vi "Scanner.vi"() -> ()   [LabVIEW 2013]
uses:
  Database/Database.lvclass
  Image/Image.lvclass
panel:
  in  "Tab Control":T1(tab)
  out "Image":T2(plugin-control)
  in  "Scan Properties":T3={"X Size"=512.0, "Y Size"=512.0, "lens"=20.0, "mag"=1.0, "Angle"=0.0}
  in  "Session":path=path "Z:/users/Manolis/Labview/Scanner/sessions_Win7.dsn"
  in  "stop":bool
  in  "x corrector":dbl=1.0
  in  "y corrector":dbl=1.0
  in  "condition":string
  out "Scan Clusters":T4(array[cluster])
  out "Vessel Cluster":T5
  out "iDatabase":i32
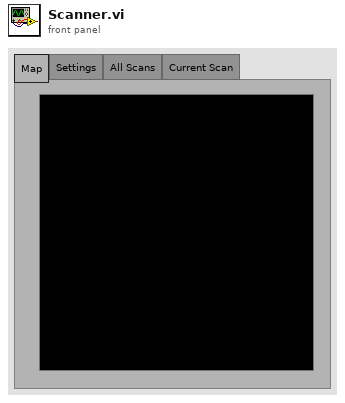
[diagram p1: front panel]
types:
  T1 = enum32{"Map", "Settings", "All Scans", "Current Scan"}
  T2 = typedef "IMAQ Image.ctl" = refnum<image>
  T3 = cluster{"X Size":dbl, "Y Size":dbl, "lens":dbl, "mag":dbl, "Angle":dbl}
  T4 = cluster{"scan_idx":string, "lens":string, "mag":string, "x":string, "y":string, "z":string, "scan_rotation":string, "scan_prog":string}[]
  T5 = cluster{"scan_idx":i32, "lens":i32, "mag":dbl, "x":dbl, "y":dbl, "mouse_id":i32, "exp_date":string, "file_name":string, "file_path":path}
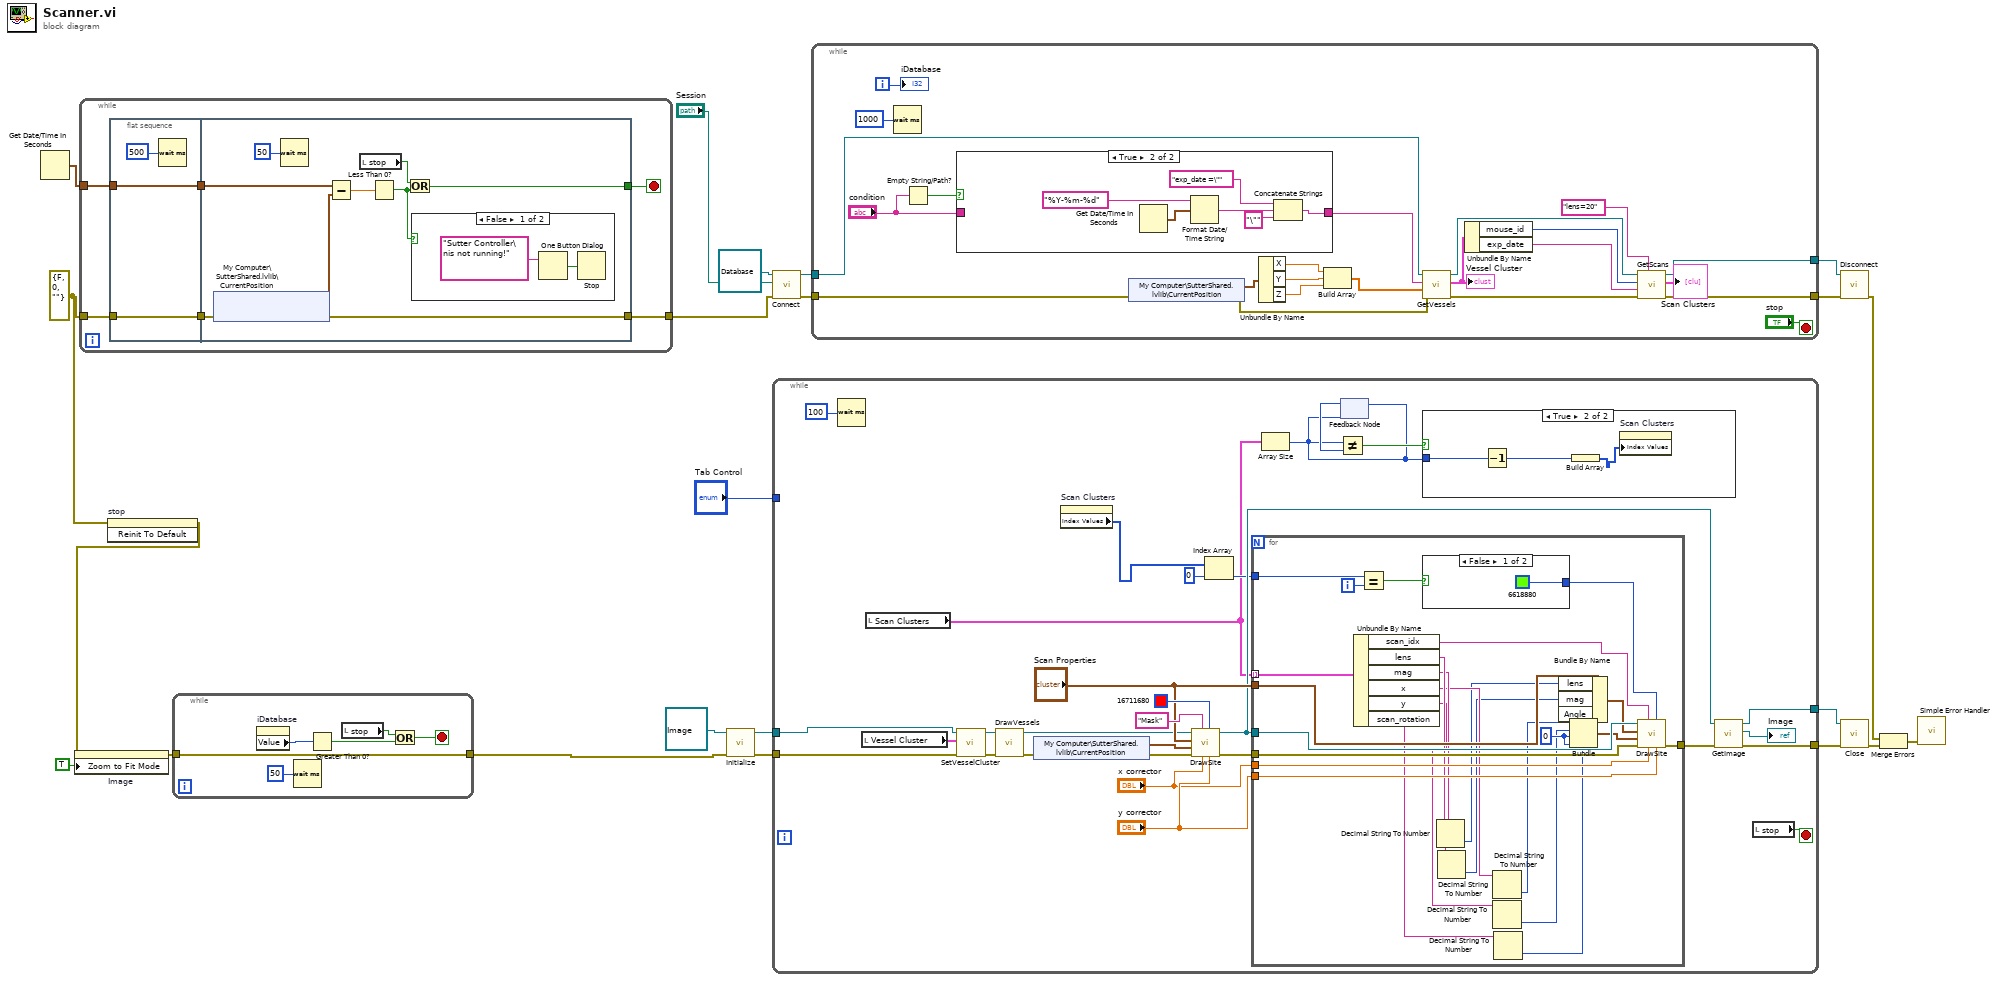
[diagram p0: block diagram]
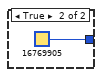
[diagram p4: hidden frame]
diagram:
  w3 = errorcluster {"status"=FALSE, "code"=0, "source"=""} ("error in (no error)")
  n1 = Get Date/Time In Seconds() -> (seconds since 1Jan1904=w5:timestamp)
  n2 = while {
    tunnel: w3 -> [w27]
    tunnel: [w26] -> w7
    tunnel: w5 -> [w25]
    stop <- w28 stop-if-true
    n3 = flat-sequence {
      tunnel: w25 -> [w30]
      tunnel: w27 -> [w31]
      tunnel: [w31] -> w24
      tunnel: [w30] -> w23
      tunnel: [w39] -> w28
      tunnel: [w36] -> w26
      tunnel: w24 -> [w37]
      tunnel: w23 -> [w34]
      frame #0 {
        n4 = Wait (ms)(milliseconds to wait=u32 500) -> ()  [unwired: 1 out]
      }
      frame #1 {
        n5 = shared-variable "My Computer\\SutterShared.lvlib\\CurrentPosition"(error in=w37) -> (error out=w36:errorcluster, w35:timestamp)  [unwired: 1 out]
        n6 = Wait (ms)(milliseconds to wait=u32 50) -> ()  [unwired: 1 out]
        n7 = Subtract(x=w34, y=w35) -> (x-y=w33:dbl)
        n8 = local read "stop"() -> (w38:bool)
        n9 = Less Than 0?(x=w33) -> (x < 0?=w32:bool)
        n10 = Or(x=w38, y=w32) -> (x .or. y?=w39:bool)
        n11 = case shown="False" w32 {
          frame False {
            n12 = One Button Dialog(message="Sutter Controller\nis not running!") -> (true=w41:bool)  [unwired: 1 in]
            n13 = Stop(stop? (T)=w41) -> ()
          }
          frame True {
          }
        }
      }
    }
  }
  n14 = invoke on="stop" class="Bool (strict)" method="Reinit To Default"(error in=w3) -> (error out=w2:errorcluster)  [unwired: 2 in, 2 out]
  n15 = property on="Image" class="ImageControl"(error in=w2, "Zoom to Fit Mode"=TRUE) -> (error out=w9:errorcluster)  [unwired: 1 in, 1 out]
  n16 = while {
    tunnel: w9 -> [w46]
    tunnel: [w46] -> w8
    stop <- w43 stop-if-true
    n17 = property on="iDatabase" class="DigNum (strict)"() -> ("Value"=w48:i32)  [unwired: 2 in, 2 out]
    n18 = Wait (ms)(milliseconds to wait=u32 50) -> ()  [unwired: 1 out]
    n19 = Greater Than 0?(x=w48) -> (x > 0?=w45:bool)
    n20 = local read "stop"() -> (w44:bool)
    n21 = Or(x=w44, y=w45) -> (x .or. y?=w43:bool)
  }
  n22 = call-dynamic "Initialize.vi"("error in (no error)"=w8, "Image in"=refnum<class "Image.lvclass"> refnum) -> ("error out"=w12:errorcluster, "Image out"=w13:refnum<class "Image.lvclass">)  [unwired: 8 in]
  n23 = call-dynamic "Connect.vi"("error in (no error)"=w7, "Session"="Session", "Database in"=refnum<class "Database.lvclass"> refnum) -> ("error out"=w19:errorcluster, "Database out"=w22:refnum<class "Database.lvclass">)  [unwired: 7 in]
  n24 = while {
    tunnel: w13 -> [w76]
    tunnel: w12 -> [w75]
    tunnel: [w74] -> w11
    tunnel: [w73] -> w10
    tunnel: "Tab Control" -> [_]
    stop <- w77 stop-if-true
    n25 = Wait (ms)(milliseconds to wait=u32 100) -> ()  [unwired: 1 out]
    n26 = local read "Vessel Cluster"() -> (w67:T5)
    n27 = local read "Scan Clusters"() -> (w57:T4)
    n28 = call-dynamic "SetVesselCluster.vi"("error in (no error)"=w75, "Vessel Cluster"=w67, "Image in"=w76) -> ("error out"=w66:errorcluster, "Image out"=w72:refnum<class "Image.lvclass">)  [unwired: 7 in]
    n29 = call-dynamic "DrawVessels.vi"("error in (no error)"=w66, "Image in"=w72) -> ("error out"=w52:errorcluster, "Image out"=w65:refnum<class "Image.lvclass">)  [unwired: 8 in]
    n30 = shared-variable "My Computer\\SutterShared.lvlib\\CurrentPosition"(error in=w52) -> (w53:cluster{"X":dbl, "Y":dbl, "Z":dbl, "Depth":dbl}, error out=w51:errorcluster)
    n31 = property on="Scan Clusters" class="Arr (strict)"() -> ("Index Values"=w50:u32[])  [unwired: 2 in, 2 out]
    n32 = call-dynamic "DrawSite.vi"("y corrector"="y corrector", "Color"=u32 16711680, "x corrector"="x corrector", "Group"="Mask", "error in (no error)"=w51, "Position"=w53, "Scan Properties"="Scan Properties", "Image in"=w65) -> ("error out"=w63:errorcluster, "Image out"=w64:refnum<class "Image.lvclass">)  [unwired: 2 in]
    n33 = Index Array(array=w50, index=0) -> (element=w58:u32)
    n34 = for {
      tunnel: w64 -> [w105]
      tunnel: w57 -> [w104] mode=indexing
      tunnel: "Scan Properties" -> [w103]
      tunnel: w63 -> [w100]
      tunnel: [w99] -> w62
      tunnel: "y corrector" -> [w98]
      tunnel: "x corrector" -> [w97]
      tunnel: w58 -> [w95]
      i -> [w96]
      w92 = 0
      n35 = Unbundle By Name(w104) -> ("scan_idx"=w91:string, "lens"=w90:string, "mag"=w89:string, "x"=w88:string, "y"=w87:string, "scan_rotation"=w86:string)
      n36 = Equal?(x=w95, y=w96) -> (x = y?=w94:bool)
      n37 = case shown="False" w94 {
        tunnel: [u32 6618880 ("Color") u32 16769905 ("Color")] -> w93
        frame False {
        }
        frame True {
        }
      }
      n38 = Decimal String To Number(string=w90) -> (number=w85:i32)  [unwired: 2 in, 1 out]
      n39 = Decimal String To Number(string=w89) -> (number=w84:i32)  [unwired: 2 in, 1 out]
      n40 = Decimal String To Number(string=w88) -> (number=w82:i32)  [unwired: 2 in, 1 out]
      n41 = Decimal String To Number(string=w87) -> (number=w81:i32)  [unwired: 2 in, 1 out]
      n42 = Decimal String To Number(string=w86) -> (number=w83:i32)  [unwired: 2 in, 1 out]
      n43 = Bundle By Name(cluster=w103, "lens"=w85, "mag"=w84, "Angle"=w83) -> (w102:T3)
      n44 = Bundle(w82, w81, w92, w92) -> (w101:cluster{i32, i32, i32, i32})  [unwired: 1 in]
      n45 = call-dynamic "DrawSite.vi"("y corrector"=w98, "Color"=w93, "x corrector"=w97, "Group"=w91, "error in (no error)"=w100, "Position"=w101, "Scan Properties"=w102, "Image in"=w105) -> ("error out"=w99:errorcluster)  [unwired: 2 in, 1 out]
    }
    n46 = Array Size(array=w57) -> (size(s)=w54:i32)
    n47 = feedback-in #1(w54) -> ()
    n48 = feedback #1(w54) -> (w56:i32)
    n49 = Not Equal?(x=w54, y=w56) -> (x != y?=w55:bool)
    n50 = case shown="True" w55 {
      tunnel: w54 -> [_ w80]
      frame False {
      }
      frame True {
        n51 = Decrement(x=w80) -> (x-1=w79:i32)
        n52 = Build Array(w79) -> (w78:i32[])
        n53 = property on="Scan Clusters" class="Arr (strict)"("Index Values"=w78) -> ()  [unwired: 2 in, 2 out]
      }
    }
    n54 = call-dynamic "GetImage.vi"("error in (no error)"=w62, "Image in"=w64) -> ("error out"=w73:errorcluster, "Image"=→"Image":T2, "Image out"=w74:refnum<class "Image.lvclass">)  [unwired: 7 in]
    n55 = local read "stop"() -> (w77:bool)
  }
  n56 = while {
    tunnel: w22 -> [w130]
    tunnel: [w129] -> w20
    tunnel: w19 -> [w116]
    tunnel: [w128] -> w18
    i -> [w117]
    stop <- "stop" stop-if-true
    n57 = Wait (ms)(milliseconds to wait=u32 1000) -> ()  [unwired: 1 out]
    n58 = Empty String/Path?(string/path="condition") -> (empty?=w126:bool)
    n59 = case shown="True" w126 {
      tunnel: [w131 w135] -> w124
      tunnel: "condition" -> [w131 _]
      frame False {
      }
      frame True {
        n60 = Get Date/Time In Seconds() -> (seconds since 1Jan1904=w134:timestamp)
        n61 = Format Date/Time String(time format string (%c)="%Y-%m-%d", seconds (now)=w134) -> (date/time string=w132:string)  [unwired: 1 in]
        n62 = Concatenate Strings("exp_date =\"", w132, "\"" ("string")) -> (w135:string)
      }
    }
    n63 = shared-variable "My Computer\\SutterShared.lvlib\\CurrentPosition"(error in=w116) -> (w113:cluster{"X":dbl, "Y":dbl, "Z":dbl, "Depth":dbl}, error out=w115:errorcluster)
    n64 = Unbundle By Name(w113) -> ("X"=w112:dbl, "Y"=w111:dbl, "Z"=w110:dbl)
    n65 = Build Array(w112, w111, w110) -> (w109:dbl[])
    n66 = call-dynamic "GetVessels.vi"("error in (no error)"=w115, "Position"=w109, "condition"=w124, "Database in"=w130) -> ("error out"=w122:errorcluster, "Vessel Cluster"=w119:T5, "Database out"=w123:refnum<class "Database.lvclass">)  [unwired: 5 in]
    "Vessel Cluster" <- w119
    n67 = Unbundle By Name(w119) -> ("mouse_id"=w121:i32, "exp_date"=w120:string)
    n68 = call-dynamic "GetScans.vi"("condition"="lens=20", "error in (no error)"=w122, "exp_date"=w120, "mouse_id"=w121, "Database in"=w123) -> ("error out"=w128:errorcluster, "Scan Clusters"=→"Scan Clusters":T4, "Database out"=w129:refnum<class "Database.lvclass">)  [unwired: 2 in, 1 out]
    "iDatabase" <- w117
  }
  n69 = call-dynamic "Disconnect.vi"("error in (no error)"=w18, "Database in"=w20) -> ("error out"=w6:errorcluster)  [unwired: 8 in, 1 out]
  n70 = call-dynamic "Close.vi"("error in (no error)"=w10, "Image in"=w11) -> ("error out"=w16:errorcluster)  [unwired: 8 in, 1 out]
  n71 = Merge Errors(w6, w16) -> (w15:errorcluster)
  n72 = call <vilib>:"Simple Error Handler.vi"("error in (no error)"=w15) -> ()  [unwired: 4 in, 5 out]
